vi "ColorMap_insidePipe.vi"(0 "Shape":cluster{"X":dbl[], "Y":dbl[]}, 1 "RedFactor":dbl, 2 "Yin":dbl, 3 "Xin":dbl) -> (5 "Inside":bool, 6 "Yout":dbl, 7 "Xout":dbl)   [LabVIEW 2016]
uses:
  <vilib>/Analysis/geometry.llb/Point in Polygon Position.ctl
  <vilib>/Analysis/geometry.llb/Point in Polygon (Scalar).vi
  <vilib>/Analysis/NI_AAL_Geometry.lvlib
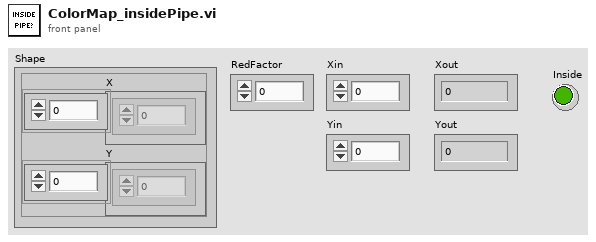
[diagram p1: front panel]
types:
  T1 = typedef "NI_AAL_Geometry.lvlib/Point in Polygon Position.ctl" = u16
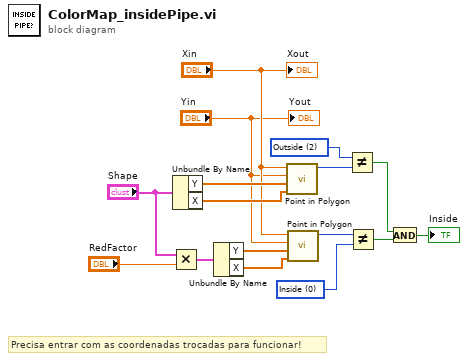
[diagram p0: block diagram]
diagram:
  w4 = T1 0 items=["Inside", "On Boundary", "Outside"] ("x")
  w6 = T1 2 items=["Inside", "On Boundary", "Outside"] ("x")
  # "Precisa entrar com as coordenadas trocadas para funcionar!"
  n1 = Multiply(x="Shape", y="RedFactor") -> (x*y=w14:cluster{"X":dbl[], "Y":dbl[]})
  n2 = Unbundle By Name("Shape") -> ("Y"=w13:dbl[], "X"=w12:dbl[])
  n3 = Unbundle By Name(w14) -> ("Y"=w11:dbl[], "X"=w10:dbl[])
  n4 = call-poly <vilib>:"Point in Polygon.vi"("Polygon Y"=w12, "Polygon X"=w13, "y"="Yin", "x"="Xin") -> ("position"=w7:T1)  [unwired: 6 in, 1 out]
  n5 = call-poly <vilib>:"Point in Polygon.vi"("Polygon Y"=w10, "Polygon X"=w11, "y"="Yin", "x"="Xin") -> ("position"=w5:T1)  [unwired: 6 in, 1 out]
  n6 = Not Equal?(x=w6, y=w7) -> (x != y?=w2:bool)
  n7 = Not Equal?(x=w5, y=w4) -> (x != y?=w3:bool)
  n8 = And(x=w2, y=w3) -> (x .and. y?=→"Inside":bool)
  "Xout" <- "Xin"
  "Yout" <- "Yin"
